vi "Fetch All Package Names.vi"(8 "error in (no error)":errorcluster) -> (0 "error out":errorcluster, 3 "All Packages":T1[](array[typedef]))   [LabVIEW 2016, in "Packages.lvlib" / "GPM.lvlib"]
uses:
  GPM.lvlib
  Package--cluster.ctl
  <vilib>/addons/JSON API/JSON Value/Set from JSON string.vi
  <vilib>/addons/database/Connection.llb/DB Tools Open Connec (String).vi
  <vilib>/addons/JSON API/JSON Scalar/Get as Text.vi
  <vilib>/addons/database/_DB Variant To Data/Database Variant To Data.xnode
  <vilib>/addons/JSON API/JSON Value/JSON Value.lvclass
  <vilib>/addons/database/NI_Database_API.lvlib
  Packages.lvlib
  <vilib>/httpClient/LabVIEWHTTPClient.lvlib
  <vilib>/addons/JSON API/Get Polymorphic/JSON GetSet.lvlib
  <vilib>/addons/JSON API/JSON Array/JSON Array.lvclass
  <vilib>/addons/JSON API/JSON Scalar/JSON Scalar.lvclass
panel:
  out "Progress":u8(slide) scale=0.0..100.0
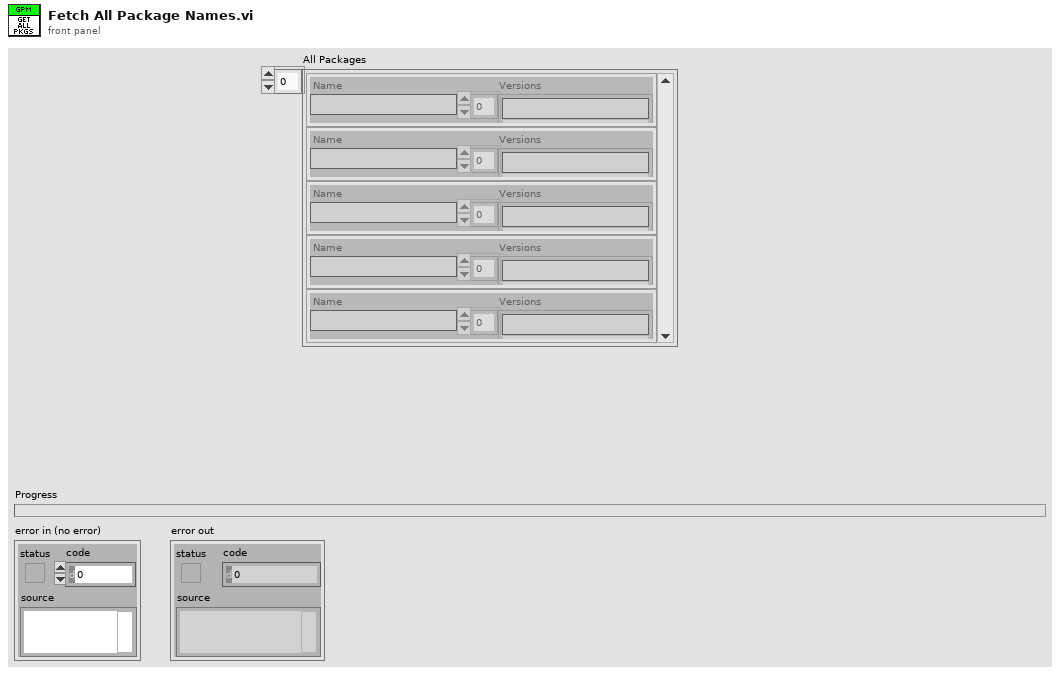
[diagram p1: front panel]
types:
  T1 = typedef "Packages.lvlib/Package--cluster.ctl" = cluster{"Name":string, "Versions":string[]}
  T2 = typedef "NI_Database_API.lvlib/Conn ObjectReference.ctl" = refnum<k1>
  T3 = typedef "LabVIEWHTTPClient.lvlib/ClientHandle.ctl" = refnum<k1>
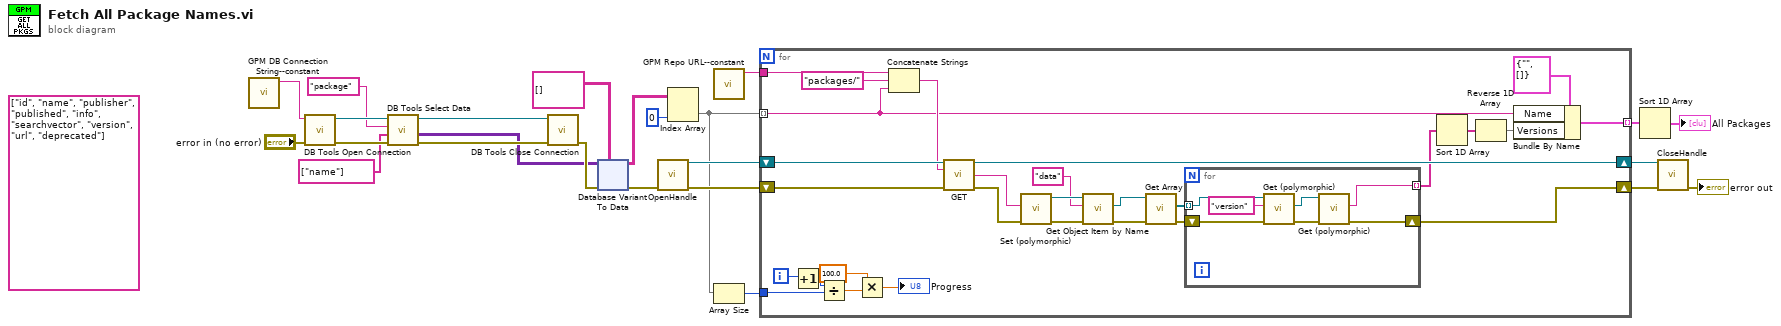
[diagram p0: block diagram]
diagram:
  (unwired) string[] ["id", "name", "publisher", "published", "info", "searchvector", "version", "url", "deprecated"] ("columns")
  n1 = call "GPM DB Connection String--constant.vi"() -> ("DB Connection String"=w24:string)  [unwired: 11 in]
  n2 = call-poly <vilib>:"DB Tools Open Connection.vi"("error in (no error)"="error in (no error)", "connection information"=w24) -> ("error out"=w23:errorcluster, "connection reference"=w22:T2)  [unwired: 6 in]
  n3 = call <vilib>:"DB Tools Select Data.vi"("error in (no error)"=w23, "columns"=string[] ["name"], "table"="package", "connection reference"=w22) -> ("error out"=w19:errorcluster, "data"=w17:variant[][], "connection reference out"=w20:T2)  [unwired: 2 in]
  n4 = call <vilib>:"DB Tools Close Connection.vi"("error in (no error)"=w19, "connection reference"=w20) -> ("error out"=w18:errorcluster)  [unwired: 5 in]
  n5 = xnode "Database Variant To Data"("database variant"=w17, "error in (no error)"=w18, "type"=string[][] []) -> ("data"=w13:string[][], "error out"=w15:errorcluster)
  n6 = call <vilib>:"OpenHandle.vi"("error in (no error)"=w15) -> ("client handle out"=w10:T3, "error out"=w11:errorcluster)  [unwired: 13 in]
  n7 = Index Array(array=w13, index (col)=0 ("disabled index (col)")) -> (element=w7:string[])  [unwired: 1 in]
  n8 = call "GPM Repo URL--constant.vi"() -> ("GPM Repo URL"=w1:string)  [unwired: 11 in]
  n9 = Array Size(array=w7) -> (size(s)=w6:i32)
  n10 = for {
    shift-right: [w39] -> w8
    shift-left: w11 -> [w52]
    tunnel: w7 -> [w35] mode=indexing
    shift-right: [w48] -> w9
    shift-left: w10 -> [w50]
    tunnel: w6 -> [w42]
    tunnel: [w31] -> w5 mode=indexing
    tunnel: w1 -> [w25]
    i -> [w43]
    n11 = Increment(x=w43) -> (x+1=w47:i32)
    n12 = Divide(x=w47, y=w42) -> (x/y=w46:dbl)
    n13 = Multiply(x=100.0, y=w46) -> (x*y=→"Progress":dbl)
    n14 = Concatenate Strings(w25, "packages/" ("string"), w35) -> (w49:string)
    n15 = call <vilib>:"GET.vi"("client handle"=w50, "url"=w49, "error in (no error)"=w52) -> ("client handle out"=w48:T3, "body"=w37:string, "error out"=w51:errorcluster)  [unwired: 9 in, 1 out]
    n16 = call-poly <vilib>:"Set (polymorphic).vi"("error in (no error)"=w51, "JSON stream"=w37) -> ("error out"=w41:errorcluster, "JSON Value out"=w29:refnum<class "JSON Value.lvclass">)  [unwired: 7 in, 1 out]
    n17 = call <vilib>:"Get Object Item by Name.vi"("error in (no error)"=w41, "name"="data", "JSON Value In"=w29) -> ("error out"=w30:errorcluster, "Value"=w27:refnum<class "JSON Value.lvclass">)  [unwired: 5 in, 2 out]
    n18 = call <vilib>:"Get Array.vi"("error in (no error)"=w30, "JSON Array in"=w27) -> ("error out"=w40:errorcluster, "Array"=w38:refnum<class "JSON Value.lvclass">[])  [unwired: 7 in, 1 out]
    n19 = for {
      shift-right: [w55] -> w39
      shift-left: w40 -> [w59]
      tunnel: w38 -> [w57] mode=indexing
      tunnel: [w53] -> w34 mode=indexing
      n20 = call-poly <vilib>:"Get (polymorphic).vi"("error in (no error)"=w59, "name"="version", "JSON Value In"=w57) -> ("error out"=w58:errorcluster, "Value"=w54:refnum<class "JSON Value.lvclass">)  [unwired: 5 in, 2 out]
      n21 = call-poly <vilib>:"Get (polymorphic).vi"("error in (no error)"=w58, "JSON Scalar in"=w54) -> ("error out"=w55:errorcluster, "LabVIEW Text"=w53:string)  [unwired: 7 in, 1 out]
    }
    n22 = Sort 1D Array(array=w34) -> (sorted array=w33:string[])
    n23 = Reverse 1D Array(array=w33) -> (reversed array=w32:string[])
    n24 = Bundle By Name(cluster=T1 {"Name"="", "Versions"=[]} ("Package"), "Name"=w35, "Versions"=w32) -> (w31:T1)
  }
  n25 = Sort 1D Array(array=w5) -> (sorted array=→"All Packages":T1[])
  n26 = call <vilib>:"CloseHandle.vi"("client handle"=w9, "error in (no error)"=w8) -> ("error out"=→"error out":errorcluster)  [unwired: 13 in]
